vi "SetDropInfo__slk_mt.vi"(8 "error in (no error)":errorcluster, 10 "drop tag":string, 11 "tree view in":refnum<class "TreeView__slk_mt.lvclass">) -> (0 "error out":errorcluster, 3 "tree view out":refnum<class "TreeView__slk_mt.lvclass">)   [LabVIEW 2020, in "TreeView__slk_mt.lvclass"]
doc: "Sets drop information."
uses:
  TreeView__slk_mt.lvclass
  TreeView__slk_mt.lvclass/TreeView__slk_mt.ctl
panel:
  # "SetDropInfo__slk_mt.vi\nSets drop information.\n\nNOTICE -- YOU MUST LEAVE THIS NOTICE IN PLACE.\n\nCopyright (c) 2011, LIANG LIU Shawn.Liu.cn@gmail.com\nAll rights reserved.\n\nRedistribution and use in source and binary forms, with or without modification, are permitted provided that the following conditions are met:\n-Redistributions of source code must retain the above copyright notice, this list of conditions and the following disclaimer.\n-Redistributions in binary form must reproduce the above copyright notice, this list of conditions and the following disclaimer in the documentation and/or other materials provided with the distribution.\n-Neither the name of the eLp nor the names of its contributors may be used to endorse or promote products derived from this software without specific prior written permission.\n\nTHIS SOFTWARE IS PROVIDED BY THE COPYRIGHT HOLDERS AND CONTRIBUTORS \"AS IS\" AND ANY EXPRESS OR IMPLIED WARRANTIES, INCLUDING, BUT NOT LIMITED TO, THE IMPLIED WARRANTIES OF MERCHANTABILITY AND FITNESS FOR A PARTICULAR PURPOSE ARE DISCLAIMED. IN NO EVENT SHALL THE COPYRIGHT HOLDER OR CONTRIBUTORS BE LIABLE FOR ANY DIRECT, INDIRECT, INCIDENTAL, SPECIAL, EXEMPLARY, OR CONSEQUENTIAL DAMAGES (INCLUDING, BUT NOT LIMITED TO, PROCUREMENT OF SUBSTITUTE GOODS OR SERVICES; LOSS OF USE, DATA, OR PROFITS; OR BUSINESS INTERRUPTION) HOWEVER CAUSED AND ON ANY THEORY OF LIABILITY, WHETHER IN CONTRACT, STRICT LIABILITY, OR TORT (INCLUDING NEGLIGENCE OR OTHERWISE) ARISING IN ANY WAY OUT OF THE USE OF THIS SOFTWARE, EVEN IF ADVISED OF THE POSSIBILITY OF SUCH DAMAGE."
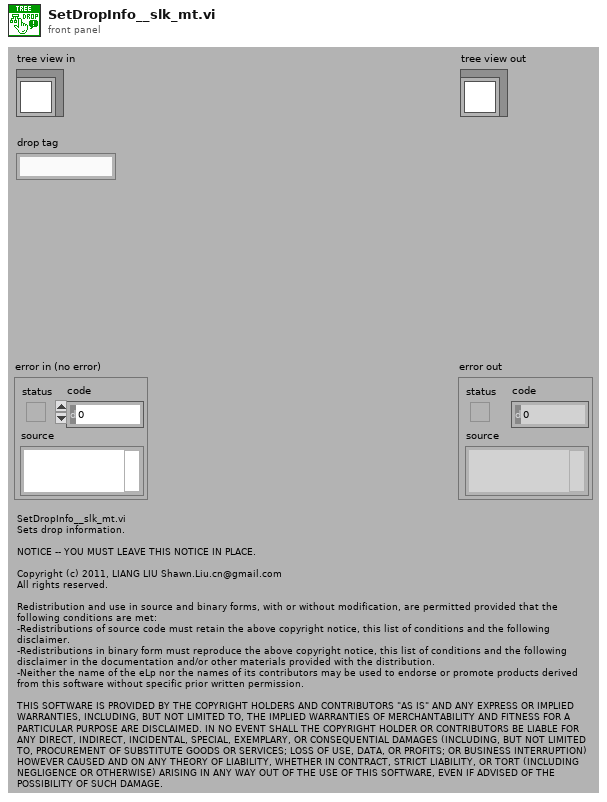
[diagram p1: front panel]
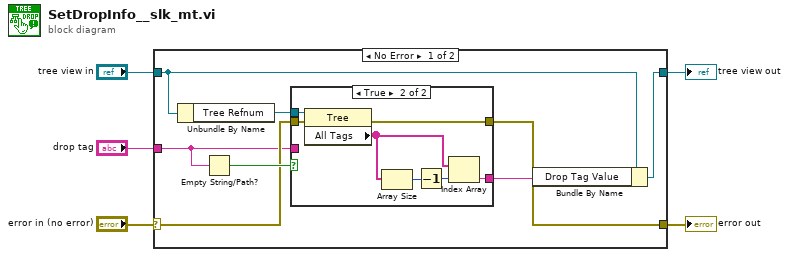
[diagram p0: block diagram]
diagram:
  n1 = case shown="No Error" "error in (no error)" {
    selector: "error in (no error)" -> [w7 w24]
    tunnel: [w8 w24] -> w4
    tunnel: [w11 w23] -> w2
    tunnel: "tree view in" -> [w9 w23]
    tunnel: "drop tag" -> [w6 _]
    frame No Error {
      n2 = Unbundle By Name(w9) -> ("Tree Refnum"=w10:refnum<vi>)
      n3 = Empty String/Path?(string/path=w6) -> (empty?=w13:bool)
      n4 = case shown="True" w13 {
        tunnel: w10 -> [_ w22]
        tunnel: [w15 w21] -> w12
        tunnel: w6 -> [w15 _]
        tunnel: w7 -> [w14 w20]
        tunnel: [w14 w16] -> w8
        frame False {
        }
        frame True {
          n5 = property class="Tree"(reference=w22, error in=w20) -> (error out=w16:errorcluster, "All Tags"=w19:string[])  [unwired: 1 out]
          n6 = Array Size(array=w19) -> (size(s)=w18:i32)
          n7 = Decrement(x=w18) -> (x-1=w17:i32)
          n8 = Index Array(array=w19, index=w17) -> (element=w21:string)
        }
      }
      n9 = Bundle By Name(cluster=w9, "Drop Tag Value"=w12) -> (w11:refnum<class "TreeView__slk_mt.lvclass">)
    }
    frame Error {
    }
  }
  "error out" <- w4
  "tree view out" <- w2
